vi "fgv_UI_ref.vi"(7 "cmd":enum16{"write", "read"}(ring), 11 "ui ref":T1) -> (3 "ui ref out":T1)   [LabVIEW 2016]
uses:
  Ctrls/ui ctrl ref2.ctl
panel:
  out "error out":errorcluster caption="err out"
  in  "error in (no error)":errorcluster caption="err in"
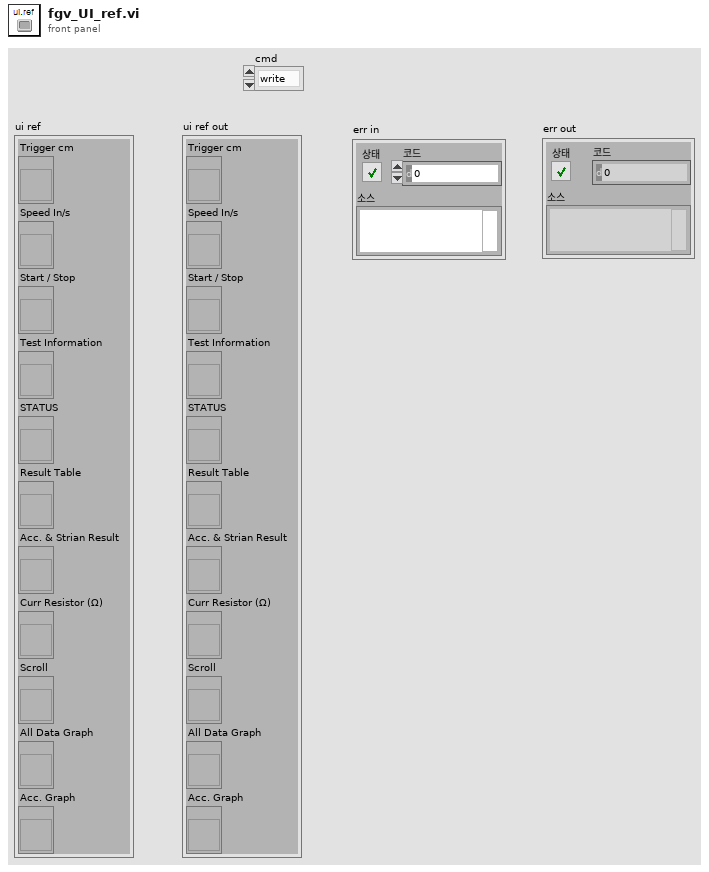
[diagram p1: front panel]
types:
  T1 = typedef "ui ctrl ref2.ctl" = cluster{"Trigger cm":refnum<vi>, "Speed In/s":refnum<vi>, "Start / Stop":refnum<vi>, "Test Information":refnum<vi>, "STATUS":refnum<vi>, "Result Table":refnum<vi>, "Acc. & Strian Result":refnum<vi>, "Curr Resistor (Ω)":refnum<vi>, "Scroll":refnum<vi>, "All Data Graph":refnum<vi>, "Acc. Graph":refnum<vi>}
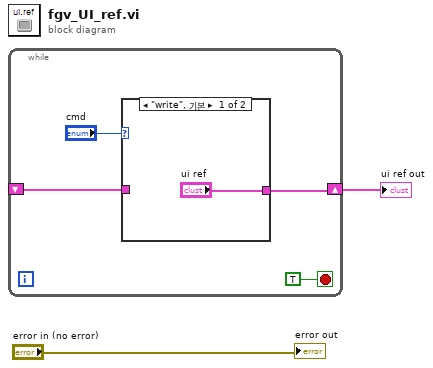
[diagram p0: block diagram]
diagram:
  n1 = while {
    shift-right: [w4] -> w1
    shift-left: _ -> [w3]
    stop <- TRUE stop-if-true
    n2 = case shown="\"write\", 기본" "cmd" {
      tunnel: ["ui ref" w8] -> w4
      tunnel: w3 -> [_ w8]
      frame "write", Default {
      }
      frame "read" {
      }
    }
  }
  "ui ref out" <- w1
  "error out" <- "error in (no error)"
